vi "Rotate90(8 bit CounterClockwise).vi"(8 "错误输入":errorcluster, 11 "image data in":T1 caption="图像数据") -> (0 "错误输出":errorcluster, 3 "image data out":T1 caption="图像数据")   [LabVIEW 2012, in "Picture Box Tools.lvlib"]
uses:
  <vilib>/picture/picture.llb/imagedata.ctl
  Picture Box Tools.lvlib
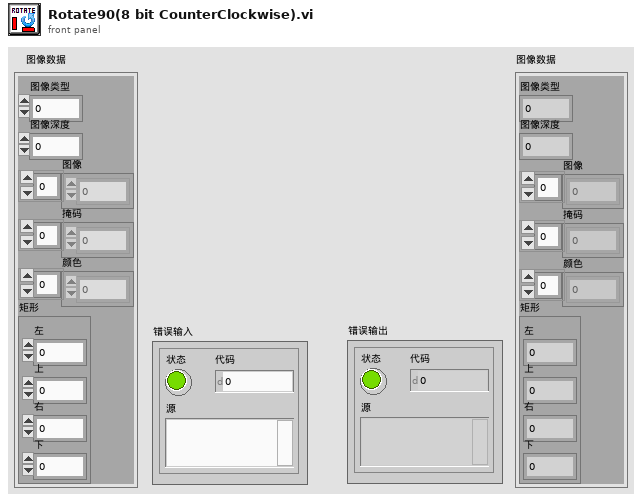
[diagram p1: front panel]
types:
  T1 = typedef "imagedata.ctl" = cluster{"image type":i32, "image depth":i32, "image":u8[], "mask":u8[], "colors":u32[], "Rectangle":cluster{"left":i16, "top":i16, "right":i16, "bottom":i16}}
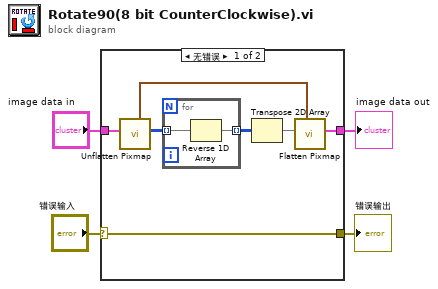
[diagram p0: block diagram]
diagram:
  n1 = case shown="无错误" "错误输入" {
    selector: "错误输入" -> [w9 w14]
    tunnel: [w9 w14] -> w3
    tunnel: "image data in" -> [w8 _]
    tunnel: [w7 _] -> w1
    frame No Error {
      n2 = call <vilib>:"Unflatten Pixmap.vi"("image data"=w8) -> ("8-bit pixmap"=w6:u8[][], "top left"=w10:cluster{"x":i16, "y":i16})  [unwired: 4 in, 5 out]
      n3 = for {
        tunnel: [w13] -> w11 mode=indexing
        tunnel: w6 -> [w12] mode=indexing
        n4 = Reverse 1D Array(array=w12) -> (reversed array=w13:u8[])
      }
      n5 = Transpose 2D Array(2D array=w11) -> (transposed array=w5:u8[][])
      n6 = call <vilib>:"Flatten Pixmap.vi"("top left"=w10, "8-bit pixmap"=w5) -> ("image data"=w7:T1)  [unwired: 9 in]
    }
    frame Error {
    }
  }
  "错误输出" <- w3
  "image data out" <- w1
